vi "testFlattenFrequencyToXML.vi"() -> ()   [LabVIEW 2012, in "UnitsAndXML.lvlib"]
uses:
  <userlib>/Common/UnitsAndXML/UnitsAndXML.lvlib
  <userlib>/Common/UnitsAndXML/FlattenItemWithUnitToXML/FlattenFrequencyToXML/FrequencyUnit.ctl
  <userlib>/Common/UnitsAndXML/FlattenItemWithUnitToXML/FlattenFrequencyToXML/typeMethods/flattenFrequencyToXML_Array.vi
  <userlib>/Common/UnitsAndXML/FlattenItemWithUnitToXML/FlattenFrequencyToXML/typeMethods/flattenFrequencyToXML_Scalar.vi
panel:
  out "error out":errorcluster
  in  "frequencyUnitInXML":T1
  out "xmlStringArray":string
  out "xmlStringScalar":string
  in  "frequency":dbl[unit][](array[numeric])=[14.999999999999998, 29.999999999999996, 45.0, 59.99999999999999]
  in  "frequency":dbl[unit]=14.999999999999998
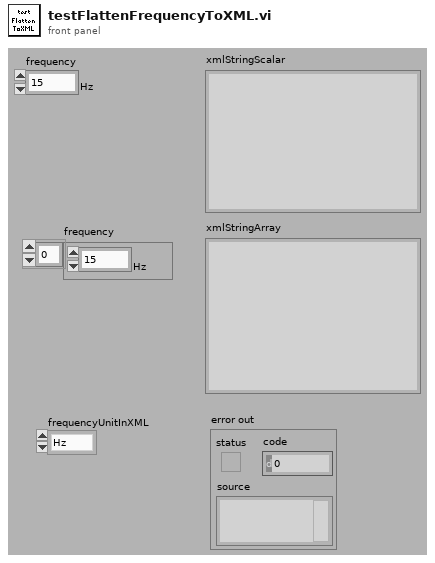
[diagram p1: front panel]
types:
  T1 = typedef "UnitsAndXML.lvlib/FrequencyUnit.ctl" = enum16{"Hz"}
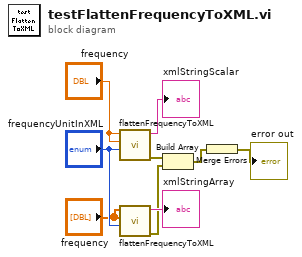
[diagram p0: block diagram]
diagram:
  n1 = call-poly <userlib>:"flattenFrequencyToXML.vi"("frequencyUnitInXML"="frequencyUnitInXML", "frequencyAgain"="frequency", "frequency"="frequency") -> ("error out"=w6:errorcluster, "xmlString"=→"xmlStringScalar":string)  [unwired: 7 in]
  n2 = call-poly <userlib>:"flattenFrequencyToXML.vi"("frequencyUnitInXML"="frequencyUnitInXML", 10:"frequency"="frequency", 11:"frequency"="frequency") -> ("error out"=w1:errorcluster, "xmlString"=→"xmlStringArray":string)  [unwired: 7 in]
  n3 = Build Array(w6, w1) -> (w7:errorcluster[])
  n4 = Merge Errors(w7) -> (→"error out":errorcluster)
